vi "Update Duration per Period.vi"(8 "error in (no error)":errorcluster, 9 "# Samples per Period":u16, 10 "Counting Gates":u16, 11 "User Interface in":refnum<class "User Interface.lvclass">) -> (0 "error out":errorcluster, 3 "User Interface out":refnum<class "User Interface.lvclass">)   [LabVIEW 2016, in "User Interface.lvlib" / "User Interface.lvclass"]
uses:
  User Interface.lvclass
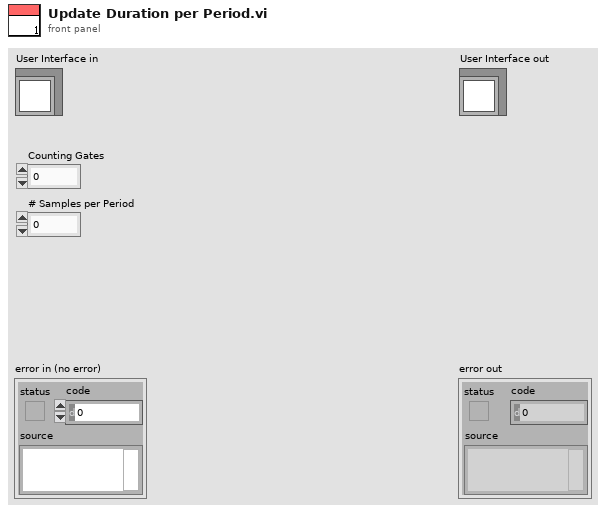
[diagram p1: front panel]
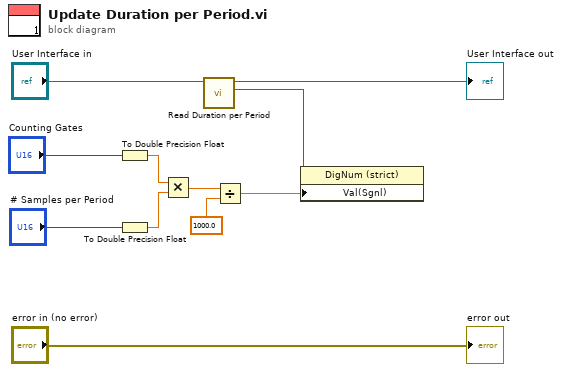
[diagram p0: block diagram]
diagram:
  n1 = To Double Precision Float(number="Counting Gates") -> (double precision float=w5:dbl)
  n2 = To Double Precision Float(number="# Samples per Period") -> (double precision float=w4:dbl)
  n3 = Multiply(x=w5, y=w4) -> (x*y=w7:dbl)
  n4 = call-dynamic "Read Duration per Period.vi"("User Interface in"="User Interface in") -> ("Duration per Period"=w3:refnum<vi>, "User Interface out"=→"User Interface out":refnum<class "User Interface.lvclass">)  [unwired: 9 in]
  n5 = Divide(x=w7, y=1000.0) -> (x/y=w2:dbl)
  n6 = property class="DigNum (strict)"(reference=w3, "Val(Sgnl)"=w2) -> ()  [unwired: 1 in, 2 out]
  "error out" <- "error in (no error)"
